vi "test - #104.vi"(8 "error in (no error)":errorcluster, 11 "TestCase in":refnum<class "testcase-Supported-Datatype.lvclass">) -> (0 "error out":errorcluster, 3 "TestCase out":refnum<class "testcase-Supported-Datatype.lvclass">)   [LabVIEW 2017, in "testcase-Supported-Datatype.lvclass"]
uses:
  testcase-Supported-Datatype.lvclass
  <vilib>/addons/_JKI Toolkits/VI Tester/TestCase.llb/TestCase.lvclass
  addons/API-String-Arugments-Support/API String Arguments Support.lvlib
  C:/Program Files (x86)/National Instruments/LabVIEW 2017/vi.lib/addons/_JKI Toolkits/VI Tester/TestCase.llb/TestCase.lvclass
panel:
  out "error out 3":errorcluster
  out "error out 2":errorcluster
  out "data 2":enum16{"MMMM", "nnnn", "ZZZZZZZ"}(ring)
  out "data":enum16{"1 - MMMM", "2 - nnnnn", "555 - QQQQQ"}(ring)
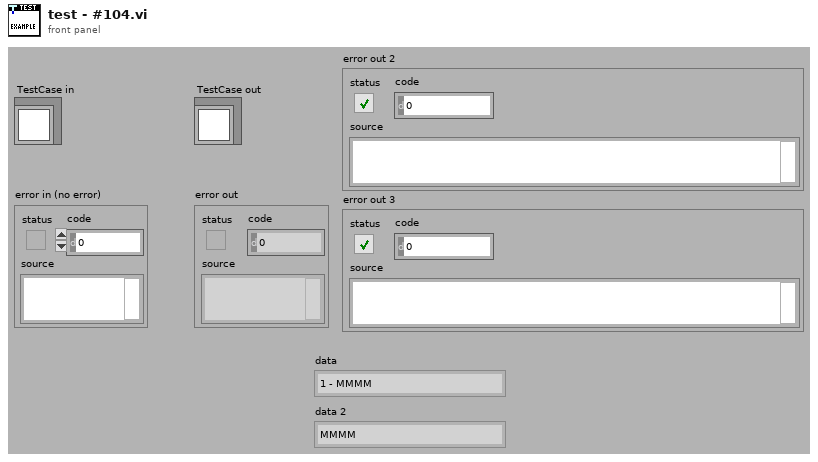
[diagram p1: front panel]
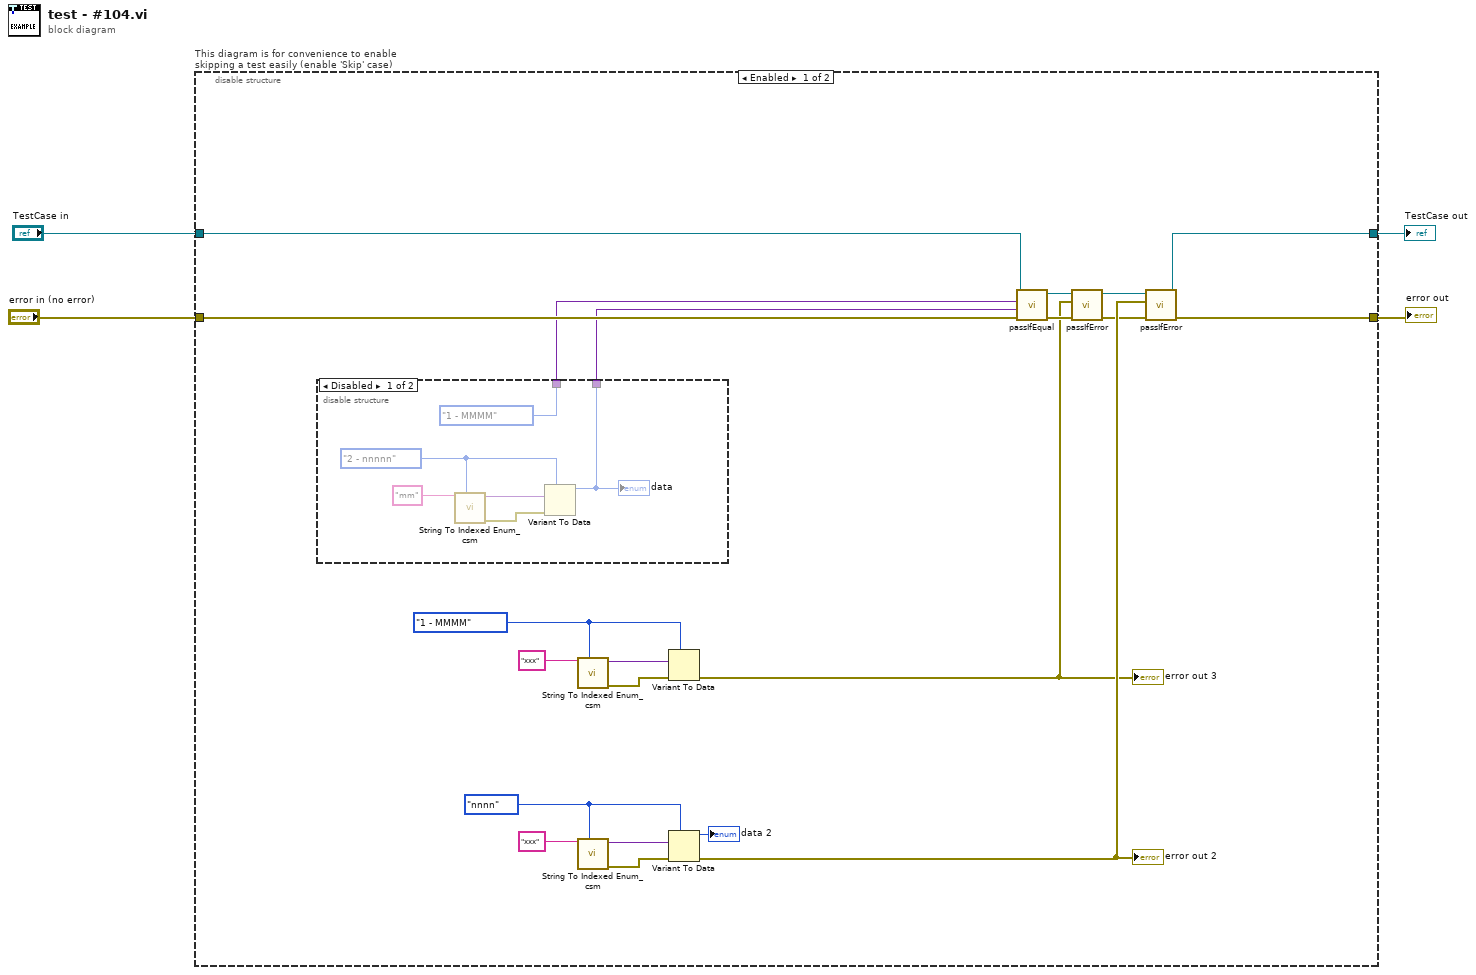
[diagram p0: block diagram]
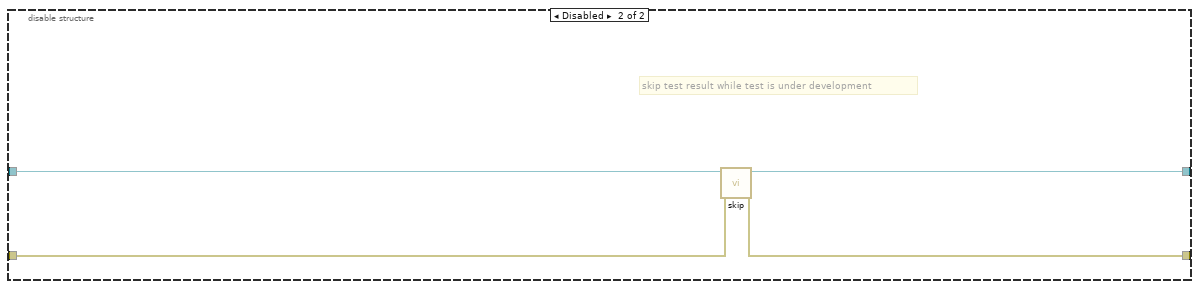
[diagram p3: hidden frame]
diagram:
  n1 = disable-structure "This diagram is for convenience to enable skipping a test easily (enable 'Skip' case)" shown="Enabled" {
    disable-tunnel: "TestCase in" -> [w25 w35]
    disable-tunnel: [w22 w33] -> w1
    disable-tunnel: [w23 w34] -> w3
    disable-tunnel: "error in (no error)" -> [w24 w32]
    frame Enabled {
      w10 = enum16{"1 - MMMM", "2 - nnnnn", "555 - QQQQQ"}."1 - MMMM" ("Data 6")
      w19 = enum16{"MMMM", "nnnn", "ZZZZZZZ"}."nnnn" ("Data 6")
      n2 = disable-structure shown="Disabled" {
        disable-tunnel: [w27 _] -> w21
        disable-tunnel: [enum16{"1 - MMMM", "2 - nnnnn", "555 - QQQQQ"}."1 - MMMM" ("Data 6") _] -> w20
        frame Disabled {
          w28 = enum16{"1 - MMMM", "2 - nnnnn", "555 - QQQQQ"}."2 - nnnnn" ("Data 6")
          n3 = call "String To Indexed Enum_csm.vi"("Variant"=w28, "String"="mm") -> ("error out"=w29:errorcluster, "Enum"=w30:variant)  [unwired: 8 in]
          n4 = Variant To Data(error in=w29, type=w28, Variant=w30) -> (data=w27:enum16{"1 - MMMM", "2 - nnnnn", "555 - QQQQQ"})  [unwired: 1 out]
          "data" <- w27
        }
        frame Enabled {
        }
      }
      n5 = call "String To Indexed Enum_csm.vi"("Variant"=w10, "String"="xxx") -> ("error out"=w11:errorcluster, "Enum"=w12:variant)  [unwired: 8 in]
      n6 = call "String To Indexed Enum_csm.vi"("Variant"=w19, "String"="xxx") -> ("error out"=w18:errorcluster, "Enum"=w17:variant)  [unwired: 8 in]
      n7 = Variant To Data(error in=w11, type=w10, Variant=w12) -> (error out=w5:errorcluster)  [unwired: 1 out]
      "error out 3" <- w5
      n8 = Variant To Data(error in=w18, type=w19, Variant=w17) -> (data=→"data 2":enum16{"MMMM", "nnnn", "ZZZZZZZ"}, error out=w15:errorcluster)
      "error out 2" <- w15
      n9 = call-dynamic "passIfEqual.vi"("error in (no error)"=w24, "y"=w21, "x"=w20, "TestCase in"=w25) -> ("error out"=w6:errorcluster, "TestCase out"=w9:refnum<class "testcase-Supported-Datatype.lvclass">)  [unwired: 6 in]
      n10 = call-dynamic "passIfError.vi"("error in (no error)"=w6, "error"=w5, "TestCase in"=w9) -> ("error out"=w7:errorcluster, "TestCase out"=w8:refnum<class "testcase-Supported-Datatype.lvclass">)  [unwired: 7 in]
      n11 = call-dynamic "passIfError.vi"("error in (no error)"=w7, "error"=w15, "TestCase in"=w8) -> ("error out"=w23:errorcluster, "TestCase out"=w22:refnum<class "testcase-Supported-Datatype.lvclass">)  [unwired: 7 in]
    }
    frame Disabled {
      # "skip test result while test is under development"
      n12 = call <vilib>:"skip.vi"("error in (no error)"=w32, "TestCase in"=w35) -> ("error out"=w34:errorcluster, "TestCase out"=w33:refnum<class "testcase-Supported-Datatype.lvclass">)  [unwired: 8 in]
    }
  }
  "error out" <- w3
  "TestCase out" <- w1
